vi "filter.vi"(9 "input":dbl) -> (1 "output":dbl)   [LabVIEW 2019]
panel:
  out "output":bool
  # "Este VI tem por objetivo filtrar os valores NaN ou INF das medições de potência, de modo a preservar a boa qualidade\ndos pontos."
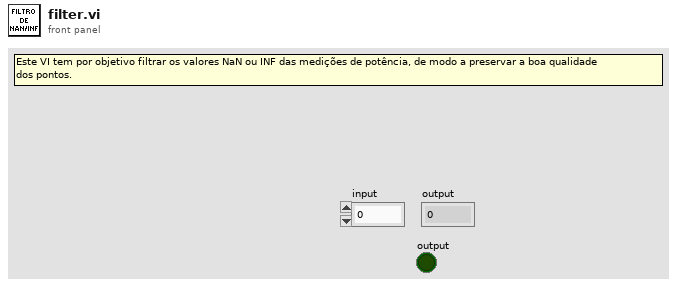
[diagram p1: front panel]
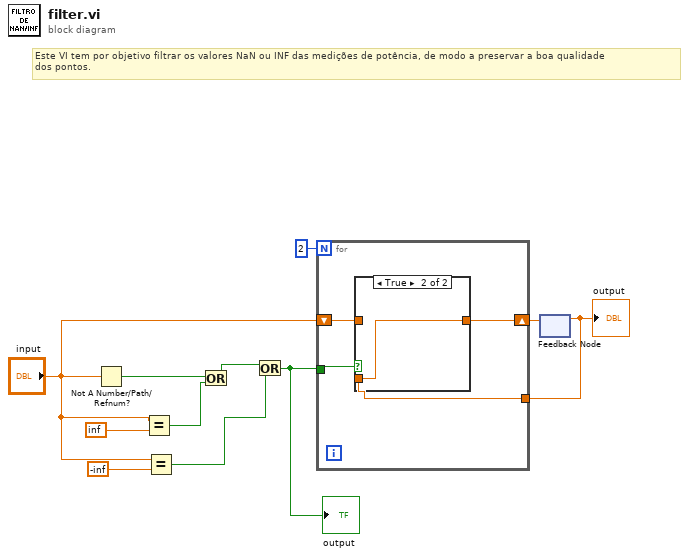
[diagram p0: block diagram]
diagram:
  # "Este VI tem por objetivo filtrar os valores NaN ou INF das medições de potência, de modo a preservar a boa qualidade\ndos pontos."
  n1 = Not A Number/Path/Refnum?(number/path/refnum="input") -> (NaN/Path/Refnum?=w11:bool)
  n2 = Equal?(x="input", y=inf) -> (x = y?=w8:bool)
  n3 = Equal?(x="input", y=-inf) -> (x = y?=w7:bool)
  n4 = Or(x=w11, y=w8) -> (x .or. y?=w4:bool)
  n5 = Or(x=w4, y=w7) -> (x .or. y?=w1:bool)
  "output" <- w1
  n6 = feedback #1() -> (w2:dbl)  [unwired: 1 in]
  "output" <- w2
  n7 = for {
    N: 2 -> [_]
    shift-right: [w14] -> w3
    shift-left: "input" -> [w13]
    tunnel: w1 -> [w15]
    tunnel: w2 -> [w12]
    n8 = case shown="True" w15 {
      tunnel: [w16 w17] -> w14
      tunnel: w13 -> [w16 _]
      tunnel: w12 -> [_ w17]
      frame False {
      }
      frame True {
      }
    }
  }
  n9 = feedback-in #1(w3) -> ()
